vi "AFT LMS IP Generator.vi"(0 "FPGA Target Refnum":refnum<vi>, 5 "Project Path":path, 7 "IP Generator Tag":string) -> ()   [LabVIEW 2017, in "NI_AdaptiveFilter.lvlib"]
uses:
  <vilib>/addons/Adaptive Filters/NI_AdaptiveFilter.lvlib
  <vilib>/addons/Adaptive Filters/Utilities/AFT Errors.ctl
panel:
  out "status":string
  in  "Load FXP Settings":bool
  out "step size maximum":dbl format="%.4g"
  out "w(n) maximum":dbl format="%.4g"
  out "d(n) maximum":dbl format="%.4g"
  out "x(n) maximum":dbl format="%.4g"
  out "close":bool
  out "Maximum input Fs@40 MHz FPGA clock":string
  in  "Help":bool
  in  "File Path":path
  in  "Read coefficients?":bool
  in  "Filter name":string="FXP LMS"
  out "step size delta":dbl format="%.4g"
  out "step size minimum":dbl format="%.4g"
  in  "step size integer word length":i32=-2 min=-128 max=128 format="%.0f bits"
  out "step size word length":i32=16 min=16 max=16 step=1 format="%.0f bits"
  in  "Step size":dbl=0.00999832 min=0.0 format="%_6g"
  in  "Filter length":i32=128 min=2 max=100000
  out "w(n) minimum":dbl format="%.4g"
  out "w(n) delta":dbl format="%.4g"
  out "d(n) minimum":dbl format="%.4g"
  out "d(n) delta":dbl format="%.4g"
  out "x(n) delta":dbl format="%.4g"
  out "x(n) minimum":dbl format="%.4g"
  in  "w(n) word length":i32(ring)=24 items=["16 bits"=16, "24 bits"=24]
  in  "d(n) word length":i32=24 min=16 max=32 step=1 format="%.0f bits"
  in  "d(n) integer word length":i32=1 min=-32 max=32 format="%.0f bits"
  in  "x(n) word length":i32=24 min=16 max=32 step=1 format="%.0f bits"
  in  "x(n) integer word length":i32=1 min=-32 max=32 format="%.0f bits"
  in  "w(n) integer word length":i32=1 min=-32 max=32 format="%.0f bits"
  in  "Cancel":bool
  in  "OK":bool
  # "Algorithm Settings"
  # "Implementation Settings"
  # "Fixed-Point Configuration"
  # "Word length"
  # "Integer word length"
  # "Minimum"
  # "Maximum"
  # "Delta"
  # "x(n)"
  # "d(n)"
  # "w(n)"
  # "Step size"
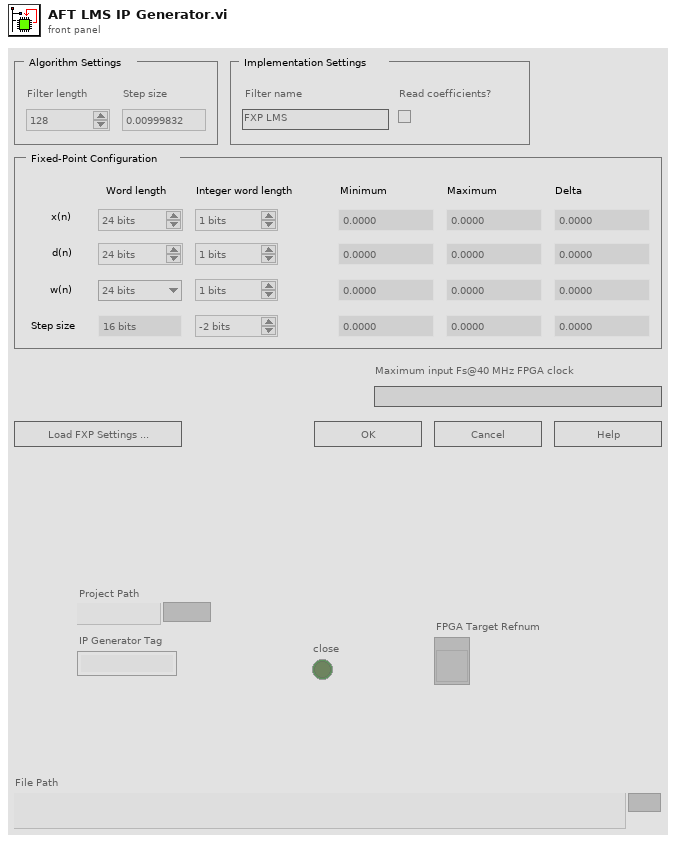
[diagram p1: front panel]
types:
  T1 = enum32{"Invalid", "Standard", "Closed", "Hidden", "Minimized", "Maximized"}
  T2 = cluster{"filter length":i32, "step size":dbl, "fixed-point configurations":cluster{"x(n) word length":i32, "x(n) integer word length":i32, "d(n) word length":i32, "d(n) integer word length":i32, "w(n) word length":i32, "w(n) integer word length":i32, "step size word length":i32, "step size integer word length":i32}}
  T3 = cluster{"x(n) word length":i32, "x(n) integer word length":i32, "d(n) word length":i32, "d(n) integer word length":i32, "w(n) word length":i32, "w(n) integer word length":i32, "step size word length":i32, "step size integer word length":i32}
  T4 = cluster{"x(n) min":dbl, "d(n) min":dbl, "w(n) min":dbl, "step size min":dbl}
  T5 = cluster{"x(n) max":dbl, "d(n) max":dbl, "w(n) max":dbl, "step size max":dbl}
  T6 = typedef "NI_AdaptiveFilter.lvlib/AFT Fixed-Point Settings.ctl" = cluster{"algorithm":u16, "filter length":i32, "step size":dbl, "encoding":cluster{"x(n) word length":i32, "x(n) integer word length":i32, "d(n) word length":i32, "d(n) integer word length":i32, "w(n) word length":i32, "w(n) integer word length":i32, "step size word length":i32, "step size integer word length":i32}}
  T7 = typedef "NI_AdaptiveFilter.lvlib/AFT Errors.ctl" = i32
  T8 = cluster{"x(n) word length":i32, "x(n) integer word length":i32, "d(n) word length":i32, "d(n) integer word length":i32, "w(n) word length":i32, "w(n) integer word length":i32, i16, "step size integer word length":i32}
  T9 = cluster{"Filter length":i32, "Step size":dbl, cluster{"x(n) word length":i32, "x(n) integer word length":i32, "d(n) word length":i32, "d(n) integer word length":i32, "w(n) word length":i32, "w(n) integer word length":i32, i16, "step size integer word length":i32}}
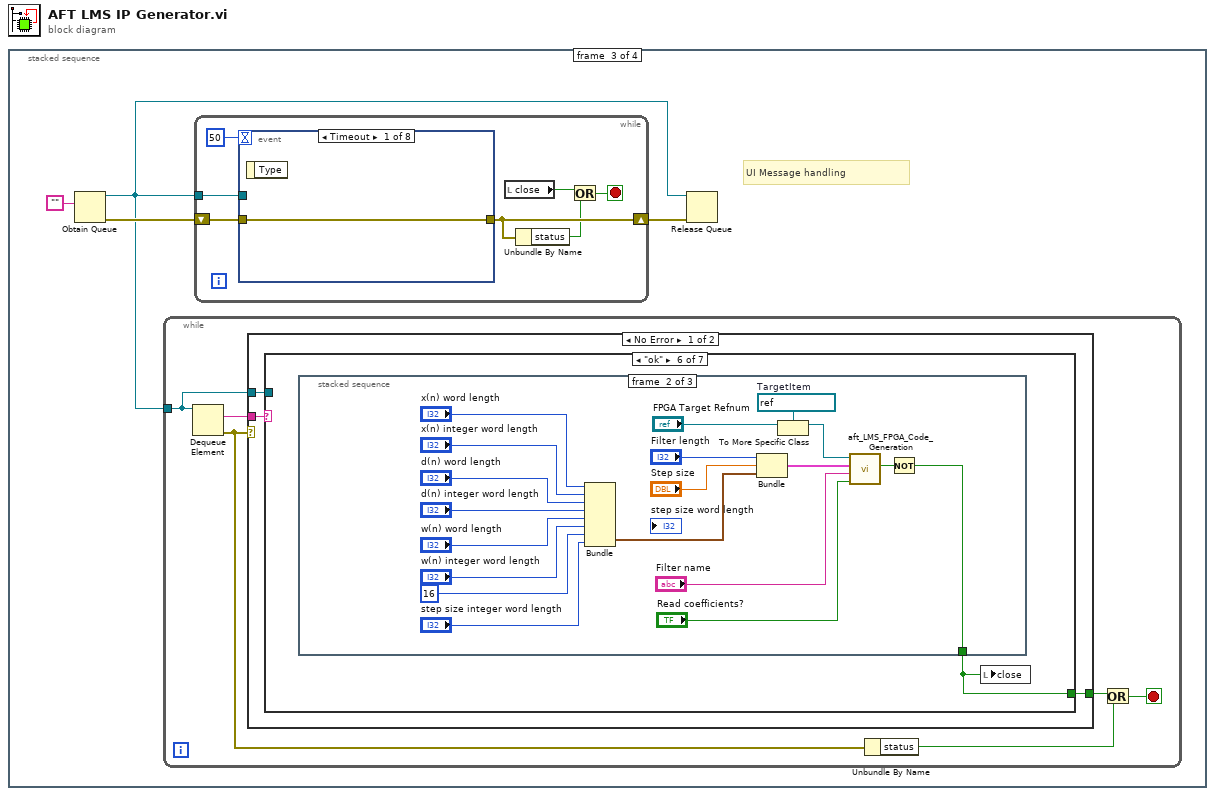
[diagram p0: block diagram]
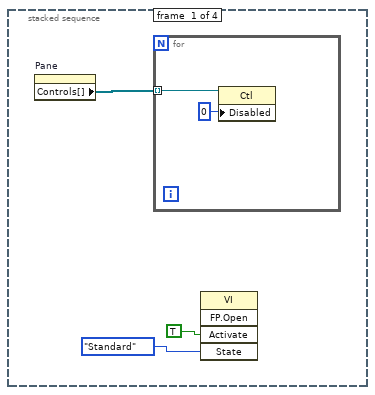
[diagram p2: hidden frame]
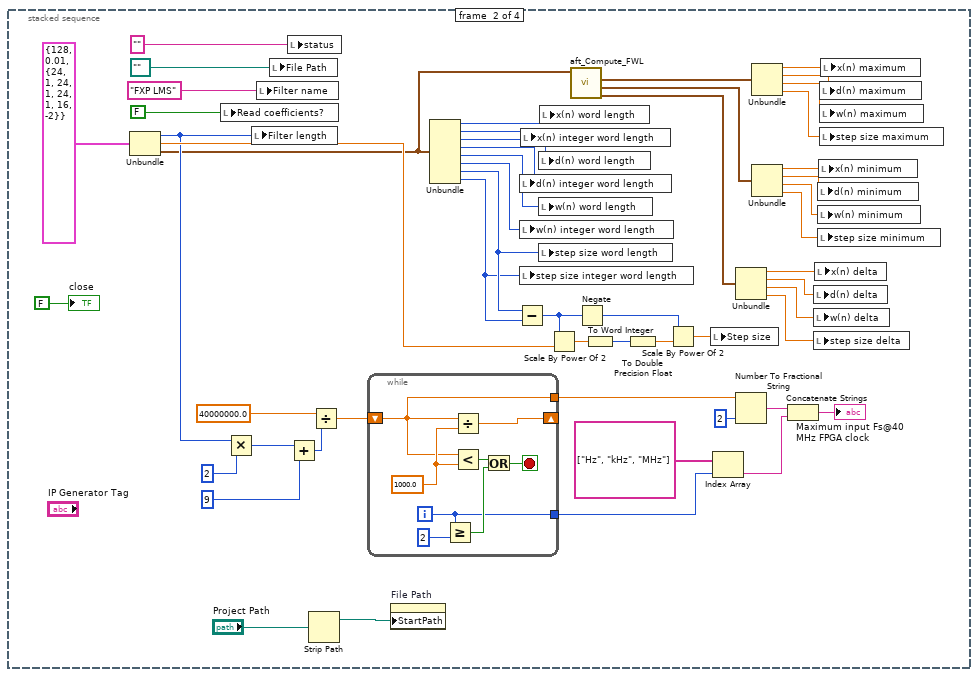
[diagram p3: hidden frame]
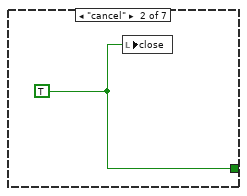
[diagram p5: hidden frame]
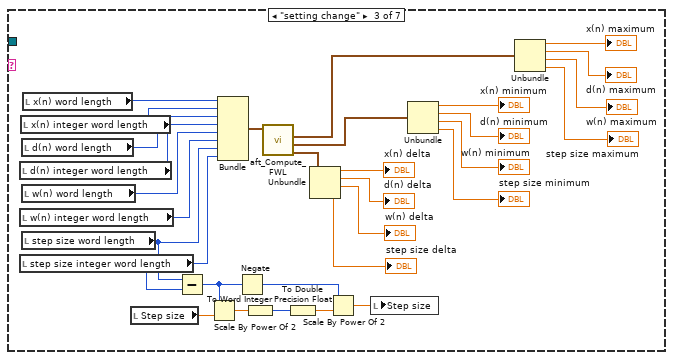
[diagram p6: hidden frame]
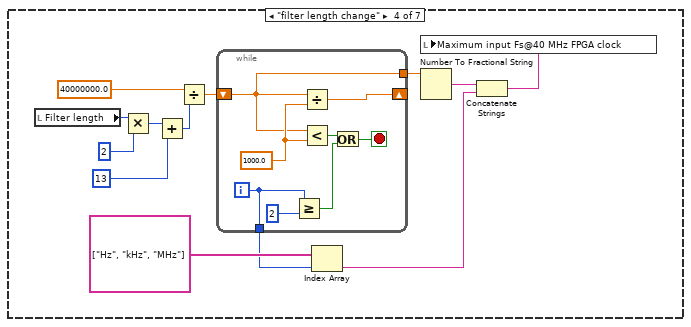
[diagram p7: hidden frame]
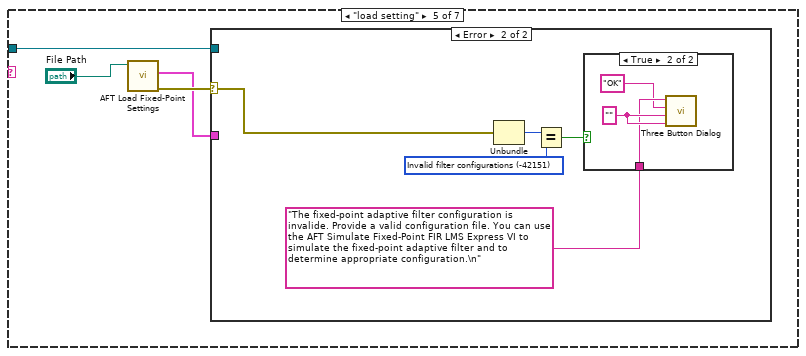
[diagram p8: hidden frame]
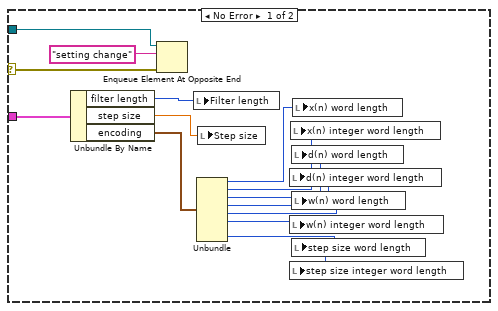
[diagram p9: hidden frame]
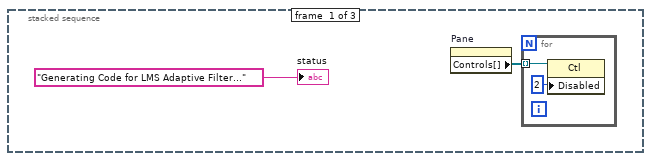
[diagram p11: hidden frame]
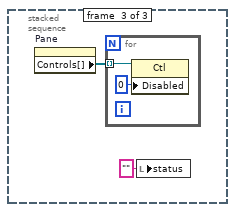
[diagram p12: hidden frame]
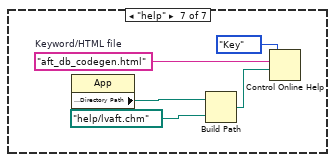
[diagram p13: hidden frame]
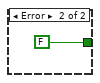
[diagram p14: hidden frame]
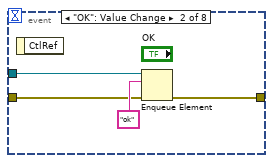
[diagram p15: hidden frame]
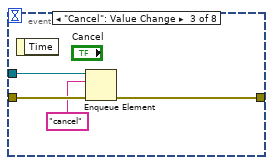
[diagram p16: hidden frame]
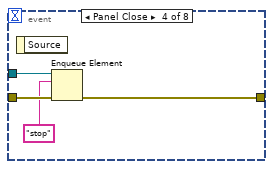
[diagram p17: hidden frame]
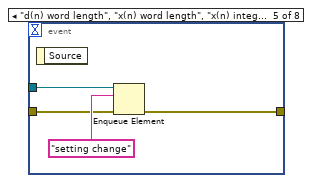
[diagram p18: hidden frame]
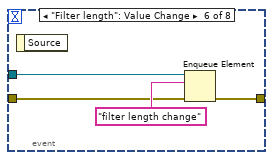
[diagram p19: hidden frame]
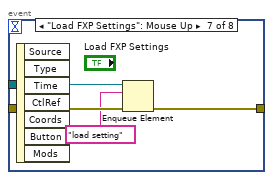
[diagram p20: hidden frame]
diagram:
  n1 = stacked-sequence {
    frame #0 {
      n2 = property on="Pane" class="Pane"() -> ("Controls[]"=w3:refnum<vi>[])  [unwired: 2 in, 2 out]
      n3 = for {
        tunnel: w3 -> [w5] mode=indexing
        n4 = property class="Ctl"(reference=w5, "Disabled"=u8 0) -> ()  [unwired: 1 in, 2 out]
      }
      n5 = invoke class="VI" method="FP.Open"("Activate"=TRUE ("Activate?"), "State"=T1."Standard") -> ()  [unwired: 3 in, 5 out]
    }
    frame #1 {
      n6 = Unbundle(T2 {"filter length"=128, "step size"=0.01, "fixed-point configurations"={"x(n) word length"=24, "x(n) integer word length"=1, "d(n) word length"=24, "d(n) integer word length"=1, "w(n) word length"=24, "w(n) integer word length"=1, "step size word length"=16, "step size integer word length"=-2}} ("fixed-point LMS settings")) -> ("filter length"=w28:i32, "step size"=w43:dbl, "fixed-point configurations"=w16:T3)
      n7 = local write "Read coefficients?"(FALSE ("Read Coefficients?")) -> ()
      n8 = Multiply(x=w28, y=2) -> (x*y=w32:i32)
      n9 = local write "Filter length"(w28) -> ()
      n10 = local write "Filter name"("FXP LMS" ("Filter Name")) -> ()
      n11 = local write "File Path"(path "" ("File Path")) -> ()
      n12 = local write "status"("" ("Status")) -> ()
      n13 = Add(x=w32, y=9) -> (x+y=w30:i32)
      n14 = Strip Path(path="Project Path") -> (stripped path=w6:path)  [unwired: 1 out]
      n15 = Divide(x=40000000.0, y=w30) -> (x/y=w27:dbl)
      n16 = while {
        shift-right: [w66] -> _
        shift-left: w27 -> [w60]
        tunnel: [w60] -> w26
        tunnel: [w59] -> w22
        i -> [w59]
        stop <- w63 stop-if-true
        w65 = 1000.0 ("y")
        n17 = Greater Or Equal?(x=w59, y=2) -> (x >= y?=w61:bool)
        n18 = Divide(x=w60, y=w65) -> (x/y=w66:dbl)
        n19 = Less?(x=w60, y=w65) -> (x < y?=w64:bool)
        n20 = Or(x=w64, y=w61) -> (x .or. y?=w63:bool)
      }
      n21 = property on="File Path" class="Path"("StartPath"=w6) -> ()  [unwired: 2 in, 2 out]
      n22 = Unbundle(w16) -> ("x(n) word length"=w42:i32, "x(n) integer word length"=w41:i32, "d(n) word length"=w40:i32, "d(n) integer word length"=w39:i32, "w(n) word length"=w38:i32, "w(n) integer word length"=w37:i32, "step size word length"=w36:i32, "step size integer word length"=w35:i32)
      n23 = Subtract(x=w36, y=w35) -> (x-y=w47:i32)
      n24 = local write "d(n) integer word length"(w39) -> ()
      n25 = local write "w(n) integer word length"(w37) -> ()
      n26 = local write "step size integer word length"(w35) -> ()
      n27 = local write "x(n) integer word length"(w41) -> ()
      n28 = local write "d(n) word length"(w40) -> ()
      n29 = local write "w(n) word length"(w38) -> ()
      n30 = local write "step size word length"(w36) -> ()
      n31 = local write "x(n) word length"(w42) -> ()
      n32 = Scale By Power Of 2(n=w47, x=w43) -> (x*2^n=w50:dbl)
      n33 = call <vilib>:"aft_Compute_FWL.vi"("fixed-point configurations"=w16) -> ("delta"=w15:cluster{dbl, dbl, dbl, dbl}, "min"=w14:T4, "max"=w13:T5)  [unwired: 8 out]
      n34 = Negate(x=w47) -> (-x=w46:i32)
      n35 = To Word Integer(number=w50) -> (16bit integer=w49:i16)
      n36 = To Double Precision Float(number=w49) -> (double precision float=w48:dbl)
      n37 = Scale By Power Of 2(n=w46, x=w48) -> (x*2^n=w45:dbl)
      n38 = local write "Step size"(w45) -> ()
      n39 = Index Array(array=string[] ["Hz", "kHz", "MHz"], index=w22) -> (element=w21:string)
      n40 = Unbundle(w15) -> (w55:dbl, w54:dbl, w53:dbl, w52:dbl)
      n41 = Number To Fractional String(number=w26, precision (6)=i16 2) -> (F-format string=w25:string)  [unwired: 2 out]
      n42 = Unbundle(w13) -> ("x(n) max"=w12:dbl, "d(n) max"=w11:dbl, "w(n) max"=w10:dbl, "step size max"=w9:dbl)
      n43 = Unbundle(w14) -> ("x(n) min"=w58:dbl, "d(n) min"=w57:dbl, "w(n) min"=w56:dbl, "step size min"=w51:dbl)
      n44 = Concatenate Strings(w25, w21) -> (→"Maximum input Fs@40 MHz FPGA clock":string)
      n45 = local write "d(n) delta"(w54) -> ()
      n46 = local write "w(n) delta"(w53) -> ()
      n47 = local write "step size delta"(w52) -> ()
      n48 = local write "x(n) delta"(w55) -> ()
      n49 = local write "d(n) minimum"(w57) -> ()
      n50 = local write "w(n) minimum"(w56) -> ()
      n51 = local write "step size minimum"(w51) -> ()
      n52 = local write "x(n) minimum"(w58) -> ()
      n53 = local write "d(n) maximum"(w11) -> ()
      n54 = local write "w(n) maximum"(w10) -> ()
      n55 = local write "step size maximum"(w9) -> ()
      n56 = local write "x(n) maximum"(w12) -> ()
      "close" <- FALSE ("close")
    }
    frame #2 {
      # "UI Message handling"
      n57 = Obtain Queue(element data type="") -> (queue out=w68:refnum<queue>, error out=w69:errorcluster)  [unwired: 3 in, 2 out]
      n58 = while {
        tunnel: w68 -> [w75]
        stop <- w72 stop-if-true
        n59 = Dequeue Element(queue=w75) -> (element=w76:string, error out=w74:errorcluster)  [unwired: 1 in, 3 out]
        n60 = case shown="No Error" w74 {
          tunnel: w76 -> [w79 _]
          tunnel: [w78 FALSE] -> w71
          tunnel: w75 -> [w77 _]
          frame No Error {
            n61 = case shown="\"ok\"" w79 {
              tunnel: [_ w80 _ _ _ w160 _] -> w78
              tunnel: w77 -> [_ _ _ _ w135 _ _]
              frame Default {
              }
              frame "cancel" {
                w80 = TRUE
                n62 = local write "close"(w80) -> ()
              }
              frame "setting change" {
                n63 = local read "d(n) integer word length"() -> (w93:i32)
                n64 = local read "w(n) integer word length"() -> (w91:i32)
                n65 = local read "step size integer word length"() -> (w89:i32)
                n66 = local read "x(n) integer word length"() -> (w95:i32)
                n67 = local read "d(n) word length"() -> (w94:i32)
                n68 = local read "w(n) word length"() -> (w92:i32)
                n69 = local read "step size word length"() -> (w90:i32)
                n70 = local read "x(n) word length"() -> (w96:i32)
                n71 = local read "Step size"() -> (w103:dbl)
                n72 = Subtract(x=w90, y=w89) -> (x-y=w99:i32)
                n73 = Scale By Power Of 2(n=w99, x=w103) -> (x*2^n=w102:dbl)
                n74 = Bundle("x(n) word length"=w96, "x(n) integer word length"=w95, "d(n) word length"=w94, "d(n) integer word length"=w93, "w(n) word length"=w92, "w(n) integer word length"=w91, "step size word length"=w90, "step size integer word length"=w89) -> (w88:T3)  [unwired: 1 out]
                n75 = Negate(x=w99) -> (-x=w98:i32)
                n76 = To Word Integer(number=w102) -> (16bit integer=w101:i16)
                n77 = call <vilib>:"aft_Compute_FWL.vi"("fixed-point configurations"=w88) -> ("delta"=w87:cluster{dbl, dbl, dbl, dbl}, "min"=w86:T4, "max"=w85:T5)  [unwired: 8 out]
                n78 = To Double Precision Float(number=w101) -> (double precision float=w100:dbl)
                n79 = Unbundle(w87) -> (→"x(n) delta":dbl, →"d(n) delta":dbl, →"w(n) delta":dbl, →"step size delta":dbl)
                n80 = Scale By Power Of 2(n=w98, x=w100) -> (x*2^n=w97:dbl)
                n81 = local write "Step size"(w97) -> ()
                n82 = Unbundle(w86) -> ("x(n) min"=→"x(n) minimum":dbl, "d(n) min"=→"d(n) minimum":dbl, "w(n) min"=→"w(n) minimum":dbl, "step size min"=→"step size minimum":dbl)
                n83 = Unbundle(w85) -> ("x(n) max"=→"x(n) maximum":dbl, "d(n) max"=→"d(n) maximum":dbl, "w(n) max"=→"w(n) maximum":dbl, "step size max"=→"step size maximum":dbl)
              }
              frame "filter length change" {
                n84 = local read "Filter length"() -> (w124:i32)
                n85 = Multiply(x=w124, y=2) -> (x*y=w122:i32)
                n86 = Add(x=w122, y=13) -> (x+y=w120:i32)
                n87 = Divide(x=40000000.0, y=w120) -> (x/y=w118:dbl)
                n88 = while {
                  shift-right: [w132] -> _
                  shift-left: w118 -> [w126]
                  tunnel: [w126] -> w115
                  tunnel: [w125] -> w116
                  i -> [w125]
                  stop <- w129 stop-if-true
                  w131 = 1000.0 ("y")
                  n89 = Greater Or Equal?(x=w125, y=2) -> (x >= y?=w127:bool)
                  n90 = Divide(x=w126, y=w131) -> (x/y=w132:dbl)
                  n91 = Less?(x=w126, y=w131) -> (x < y?=w130:bool)
                  n92 = Or(x=w130, y=w127) -> (x .or. y?=w129:bool)
                }
                n93 = Index Array(array=string[] ["Hz", "kHz", "MHz"], index=w116) -> (element=w113:string)
                n94 = Number To Fractional String(number=w115) -> (F-format string=w114:string)  [unwired: 3 out]
                n95 = Concatenate Strings(w114, w113) -> (w112:string)
                n96 = local write "Maximum input Fs@40 MHz FPGA clock"(w112) -> ()
              }
              frame "load setting" {
                n97 = call <vilib>:"AFT Load Fixed-Point Settings.vi"("file path in"="File Path") -> ("error out"=w134:errorcluster, "fixed-point settings"=w133:T6)  [unwired: 1 in, 8 out]
                n98 = case shown="Error" w134 {
                  selector: w134 -> [w141 w153]
                  tunnel: w133 -> [w140 _]
                  tunnel: w135 -> [w143 _]
                  frame No Error {
                    n99 = Unbundle By Name(w140) -> ("filter length"=w138:i32, "step size"=w137:dbl, "encoding"=w139:T3)
                    n100 = Enqueue Element At Opposite End(queue=w143, element="setting change", error in (no error)=w141) -> ()  [unwired: 4 out]
                    n101 = local write "Filter length"(w138) -> ()
                    n102 = Unbundle(w139) -> ("x(n) word length"=w151:i32, "x(n) integer word length"=w150:i32, "d(n) word length"=w149:i32, "d(n) integer word length"=w148:i32, "w(n) word length"=w147:i32, "w(n) integer word length"=w146:i32, "step size word length"=w145:i32, "step size integer word length"=w144:i32)
                    n103 = local write "Step size"(w137) -> ()
                    n104 = local write "d(n) integer word length"(w148) -> ()
                    n105 = local write "w(n) integer word length"(w146) -> ()
                    n106 = local write "step size integer word length"(w144) -> ()
                    n107 = local write "x(n) integer word length"(w150) -> ()
                    n108 = local write "d(n) word length"(w149) -> ()
                    n109 = local write "w(n) word length"(w147) -> ()
                    n110 = local write "step size word length"(w145) -> ()
                    n111 = local write "x(n) word length"(w151) -> ()
                  }
                  frame Error {
                    w155 = T7 -42151 items=["No errors"=0, "No valid FPGA target"=-42150, "Invalid filter configurations"=-42151, "LabVIEW FPGA or NI-RIO not installed"=-42152, "File exists on disk"=-42153, "File exists in memory"=-42154, "Item exists in project"=-42155, "Invalid filter name"=-42156] ("AFT errors")
                    n112 = Unbundle(w153) -> ("code"=w156:i32)  [unwired: 2 out]
                    n113 = Equal?(x=w156, y=w155) -> (x = y?=w154:bool)
                    n114 = case shown="True" w154 {
                      tunnel: "The fixed-point adaptive filter configuration is invalide. Provide a valid configuration file. You can use the AFT Simulate Fixed-Point FIR LMS Express VI to simulate the fixed-point adaptive filter and to determine appropriate configuration.\n" ("Tips") -> [_ w158]
                      frame False {
                      }
                      frame True {
                        w159 = "" ("Center Button Text (\"No\")")
                        n115 = call <vilib>:"Three Button Dialog.vi"("Right Button Text (\"Cancel\")"=w159, "Center Button Text (\"No\")"=w159, "Left Button Text (\"Yes\")"="OK" ("Left Button Text (\"Yes\")"), "message"=w158) -> ()  [unwired: 1 in, 7 out]
                      }
                    }
                  }
                }
              }
              frame "ok" {
                n116 = stacked-sequence {
                  tunnel: [_ w165 _] -> w160
                  frame #0 {
                    n117 = property on="Pane" class="Pane"() -> ("Controls[]"=w161:refnum<vi>[])  [unwired: 2 in, 2 out]
                    n118 = for {
                      tunnel: w161 -> [w164] mode=indexing
                      n119 = property class="Ctl"(reference=w164, "Disabled"=u8 2) -> ()  [unwired: 1 in, 2 out]
                    }
                    "status" <- "Generating Code for LMS Adaptive Filter..." ("Status")
                  }
                  frame #1 {
                    w181 = refnum<vi> refnum  # TargetItem
                    n120 = Bundle("x(n) word length"="x(n) word length", "x(n) integer word length"="x(n) integer word length", "d(n) word length"="d(n) word length", "d(n) integer word length"="d(n) integer word length", "w(n) word length"="w(n) word length", "w(n) integer word length"="w(n) integer word length", i16 16, "step size integer word length"="step size integer word length") -> (w179:T8)  [unwired: 1 out]
                    n121 = Bundle("Filter length"="Filter length", "Step size"="Step size", w179) -> (w180:T9)  [unwired: 1 out]
                    n122 = To More Specific Class(target class=w181, reference="FPGA Target Refnum") -> (specific class reference=w182:refnum<vi>)  [unwired: 1 in, 1 out]
                    n123 = call <vilib>:"aft_LMS_FPGA_Code_Generation.vi"("read coefficient? (F)"="Read coefficients?", "filter name"="Filter name", "fixed-point LMS settings"=w180, "target item"=w182) -> ("continue?"=w166:bool)  [unwired: 7 out]
                    n124 = Not(x=w166) -> (.not. x?=w165:bool)
                  }
                  frame #2 {
                    n125 = property on="Pane" class="Pane"() -> ("Controls[]"=w185:refnum<vi>[])  [unwired: 2 in, 2 out]
                    n126 = for {
                      tunnel: w185 -> [w187] mode=indexing
                      n127 = property class="Ctl"(reference=w187, "Disabled"=u8 0) -> ()  [unwired: 1 in, 2 out]
                    }
                    n128 = local write "status"("" ("status")) -> ()
                  }
                }
                n129 = local write "close"(w160) -> ()
              }
              frame "help" {
                w190 = "aft_db_codegen.html"  # Keyword/HTML file
                n130 = property class="App"() -> ("Application:Directory Path"=w192:path)  [unwired: 2 in, 2 out]
                n131 = Build Path(base path=w192, name or relative path=path "help/lvaft.chm") -> (appended path=w189:path)
                n132 = Control Online Help(2:w189, 3:w190, 4:enum16{"Contents", "Key", "Close"}."Key" ("Operation")) -> ()  [unwired: 1 in, 1 out]
              }
            }
          }
          frame Error {
          }
        }
        n133 = Unbundle By Name(w74) -> ("status"=w73:bool)
        n134 = Or(x=w71, y=w73) -> (x .or. y?=w72:bool)
      }
      n135 = while {
        tunnel: w68 -> [w200]
        shift-right: [w197] -> w67
        shift-left: w69 -> [w199]
        stop <- w196 stop-if-true
        n136 = event shown="[0] Timeout" {
          selector: _ -> [_ _ _ _ _ _ _ _]
          dyn-events: _ -> [_ _ _ _ _ _ _ _]
          timeout: 50 -> [_ _ _ _ _ _ _ _]
          tunnel: w200 -> [_ w203 w209 w213 w216 w220 w225 w229]
          tunnel: w199 -> [w201 w202 w208 w212 w215 w219 w224 w228]
          tunnel: [w201 w205 w207 w211 w214 w218 w223 w227] -> w197
          event Timeout {
            n137 = event-data() -> ()  [unwired: 2 out]
          }
          event "OK": Value Change {
            n138 = event-data() -> ()  [unwired: 2 out]
            n139 = Enqueue Element(queue=w203, element="ok", error in (no error)=w202) -> (error out=w205:errorcluster)  [unwired: 3 out]
          }
          event "Cancel": Value Change {
            n140 = event-data() -> ()  [unwired: 2 out]
            n141 = Enqueue Element(queue=w209, element="cancel", error in (no error)=w208) -> (error out=w207:errorcluster)  [unwired: 3 out]
          }
          event Panel Close {
            n142 = event-data() -> ()  [unwired: 2 out]
            n143 = Enqueue Element(queue=w213, element="stop", error in (no error)=w212) -> (error out=w211:errorcluster)  [unwired: 3 out]
          }
          event "d(n) word length", "x(n) word length", "x(n) integer word length", "d(n) integer word length", "w(n) integer word length", "w(n) word length", "step size word length", "step size integer word length", "Step size": Value Change {
            n144 = event-data() -> ()  [unwired: 2 out]
            n145 = Enqueue Element(queue=w216, element="setting change", error in (no error)=w215) -> (error out=w214:errorcluster)  [unwired: 3 out]
          }
          event "Filter length": Value Change {
            n146 = event-data() -> ()  [unwired: 2 out]
            n147 = Enqueue Element(queue=w220, element="filter length change", error in (no error)=w219) -> (error out=w218:errorcluster)  [unwired: 3 out]
          }
          event "Load FXP Settings": Mouse Up {
            n148 = event-data() -> ()  [unwired: 8 out]
            n149 = Enqueue Element(queue=w225, element="load setting", error in (no error)=w224) -> (error out=w223:errorcluster)  [unwired: 3 out]
          }
          event "Help": Value Change {
            n150 = event-data() -> ()  [unwired: 2 out]
            n151 = Enqueue Element(queue=w229, element="help", error in (no error)=w228) -> (error out=w227:errorcluster)  [unwired: 3 out]
          }
        }
        n152 = local read "close"() -> (w194:bool)
        n153 = Unbundle By Name(w197) -> ("status"=w195:bool)
        n154 = Or(x=w194, y=w195) -> (x .or. y?=w196:bool)
      }
      n155 = Release Queue(queue=w68, error in (no error)=w67) -> ()  [unwired: 4 out]
    }
    frame #3 {
      n156 = invoke class="VI" method="FP.Close"() -> ()  [unwired: 3 in, 3 out]
    }
  }
